vi "Channel States json test - state string.vi"() -> ()   [LabVIEW 2017, in "Switch Scripting.lvlib"]
uses:
  Switch Scripting.lvlib
  Channel States.ctl
  Routing State.ctl
  Routing Channel/Connection.ctl
panel:
  out "State names":string[](array[string])
  out "Channel States from JSON":T1=[{"name"="", "description"="", "value"=23, "connection list"=[{"source"="2010A:J1Ch0p", "destination"="2010A:J2Ch16p"}]}, {"name"="", "description"="", "value"=34, "connection list"=[{"source"="2010A:J1Ch0p", "destination"="2010A:J2Ch0p"}, {"source"="2010B:J1Ch0p", "destination"="2010B:J2Ch0p"}]}]
  out "Connection List":cluster{"Source":string, "Destination":string}[](array[cluster])
  in  "run-time Channel state":i32
  out "State values":i32[](array[numeric])
  out "JSON string":string
  in  "Channel States":T1=[{"name"="simple", "description"="", "value"=23, "connection list"=[{"source"="2010A:J1Ch0p", "destination"="2010A:J2Ch16p"}]}, {"name"="addOne", "description"="", "value"=34, "connection list"=[{"source"="2010A:J1Ch0p", "destination"="2010A:J2Ch0p"}, {"source"="2010B:J1Ch0p", "destination"="2010B:J2Ch0p"}]}]
  # "Compiled --- >>"
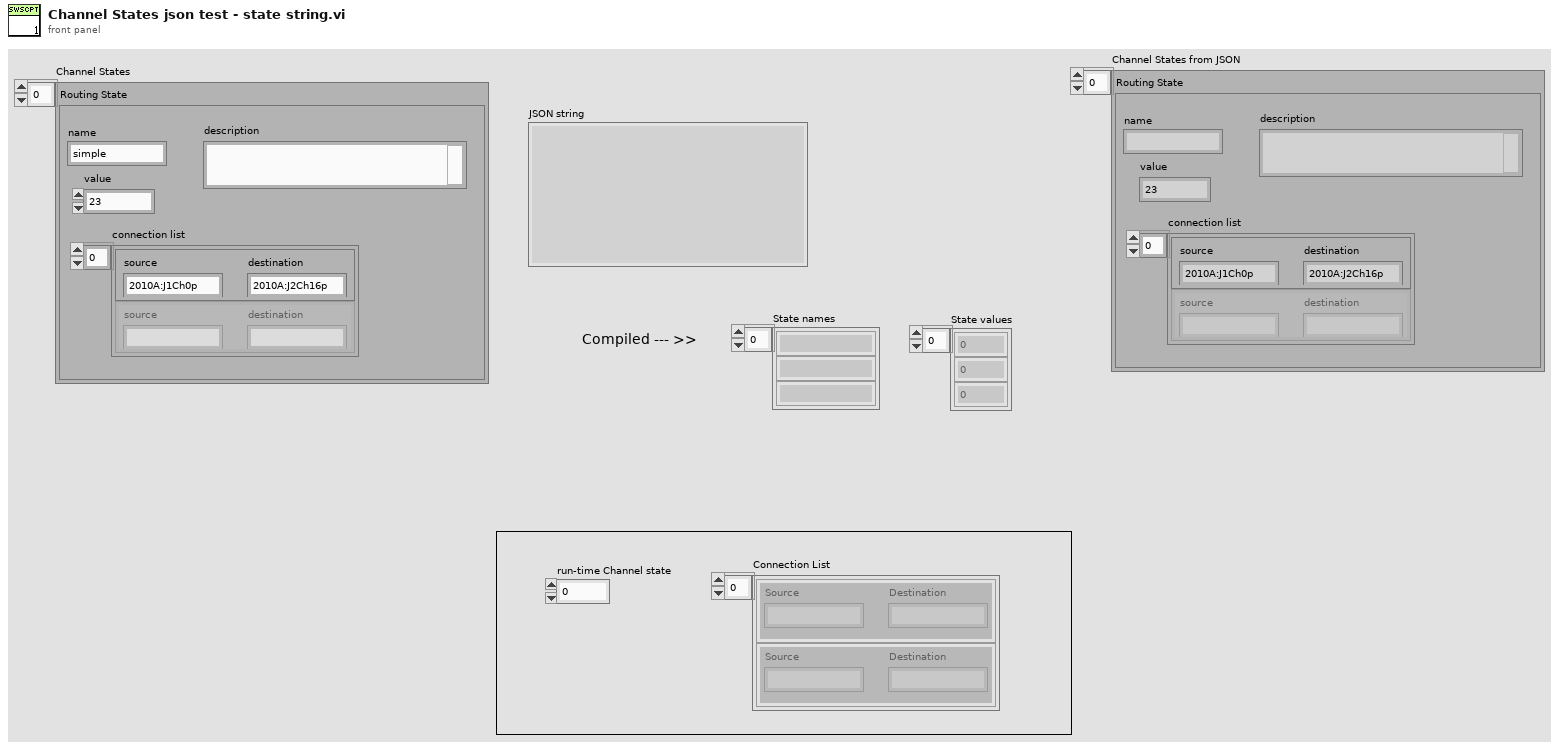
[diagram p1: front panel]
types:
  T1 = typedef "Switch Scripting.lvlib/Channel States.ctl" = T2[]
  T2 = typedef "Switch Scripting.lvlib/Routing State.ctl" = cluster{"name":string, "description":string, "value":i32, "connection list":T3[]}
  T3 = typedef "Switch Scripting.lvlib/Connection.ctl" = cluster{"source":string, "destination":string}
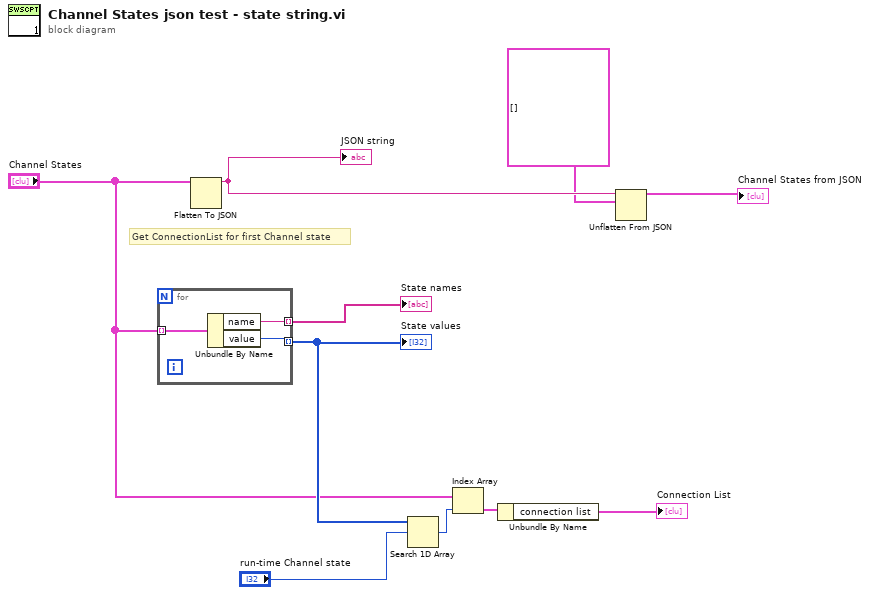
[diagram p0: block diagram]
diagram:
  # "Get ConnectionList for first Channel state"
  n1 = for {
    tunnel: "Channel States" -> [w13] mode=indexing
    tunnel: [w12] -> w9 mode=indexing
    tunnel: [w11] -> w1 mode=indexing
    n2 = Unbundle By Name(w13) -> ("name"=w11:string, "value"=w12:i32)
  }
  "State values" <- w9
  "State names" <- w1
  n3 = Flatten To JSON(anything="Channel States") -> (JSON string=w5:string)  [unwired: 2 in, 1 out]
  "JSON string" <- w5
  n4 = Search 1D Array(1D array=w9, element="run-time Channel state") -> (index of element=w7:i32)  [unwired: 1 in]
  n5 = Index Array(array="Channel States", index=w7) -> (element=w10:T2)
  n6 = Unbundle By Name(w10) -> ("connection list"=→"Connection List":T3[])
  n7 = Unflatten From JSON(JSON string=w5, type and defaults=T1 [] ("Channel States")) -> (value=→"Channel States from JSON":T1)  [unwired: 5 in, 1 out]
